vi "UnitChange.vi"(5 "Unit":T1, 11 "error in (no error)":errorcluster) -> (15 "error out":errorcluster)   [LabVIEW 2014, in "FH 55.lvlib"]
uses:
  FH 55.lvlib
  TypeDef/Unit.ctl
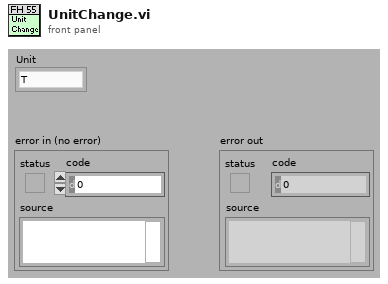
[diagram p1: front panel]
types:
  T1 = typedef "FH 55.lvlib/Unit.ctl" = enum16{"T", "G", "A/m"}
  T2 = typedef "FH 55.lvlib/Value_String.ctl" = cluster{"Numeric":dbl, "String":string}
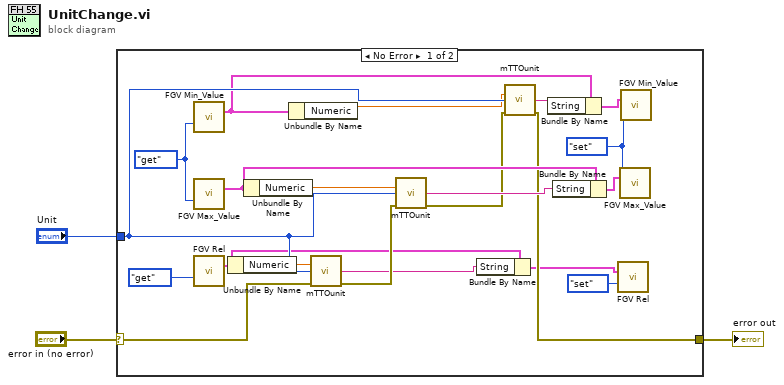
[diagram p0: block diagram]
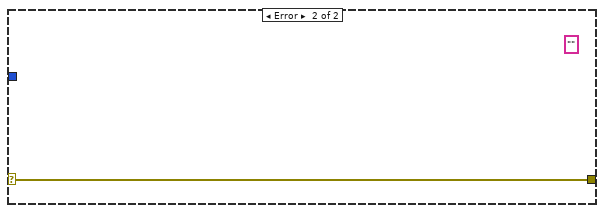
[diagram p2: hidden frame]
diagram:
  n1 = case shown="No Error" "error in (no error)" {
    selector: "error in (no error)" -> [w8 w25]
    tunnel: [w10 w25] -> w2
    tunnel: "Unit" -> [w22 _]
    frame No Error {
      w15 = enum16{"set", "get"}."set" ("action")
      w23 = enum16{"set", "get"}."get" ("action")
      n2 = call "FGV Min_Value.vi"("action"=w23) -> ("Extrem_Value 2"=w20:T2)  [unwired: 14 in]
      n3 = call "FGV Max_Value.vi"("action"=w23) -> ("Extrem_Value 2"=w19:T2)  [unwired: 14 in]
      n4 = call "FGV Rel.vi"("action"=enum16{"set", "get"}."get") -> ("Extrem_Value"=w6:T2)  [unwired: 13 in, 1 out]
      n5 = Unbundle By Name(w6) -> ("Numeric"=w7:dbl)
      n6 = Unbundle By Name(w19) -> ("Numeric"=w14:dbl)
      n7 = Unbundle By Name(w20) -> ("Numeric"=w13:dbl)
      n8 = call "mTTOunit.vi"("Numeric"=w7, "Unit"=w22, "error in (no error)"=w8) -> ("Display"=w5:string, "error out"=w12:errorcluster)  [unwired: 10 in, 1 out]
      n9 = call "mTTOunit.vi"("Numeric"=w14, "Unit"=w22, "error in (no error)"=w12) -> ("Display"=w18:string, "error out"=w11:errorcluster)  [unwired: 10 in, 1 out]
      n10 = Bundle By Name(cluster=w6, "String"=w5) -> (w4:T2)
      n11 = call "mTTOunit.vi"("Numeric"=w13, "Unit"=w22, "error in (no error)"=w11) -> ("Display"=w21:string, "error out"=w10:errorcluster)  [unwired: 10 in, 1 out]
      n12 = Bundle By Name(cluster=w20, "String"=w21) -> (w16:T2)
      n13 = Bundle By Name(cluster=w19, "String"=w18) -> (w17:T2)
      n14 = call "FGV Rel.vi"("Extrem_Value"=w4, "action"=enum16{"set", "get"}."set") -> ()  [unwired: 12 in, 2 out]
      n15 = call "FGV Max_Value.vi"("Extrem_Value"=w17, "action"=w15) -> ()  [unwired: 13 in, 1 out]
      n16 = call "FGV Min_Value.vi"("Extrem_Value"=w16, "action"=w15) -> ()  [unwired: 13 in, 1 out]
    }
    frame Error {
      (unwired) ""
    }
  }
  "error out" <- w2
